vi "joe_send_message.vi"(4 "write buffer":string, 7 "source":string, 8 "write mode (set END:0)":i32(ring) items=["send EOI with last character of string", "append CR to string and send EOI with CR", "append LF to string and send EOI with LF", "append CR LF to string and send EOI with LF", "append CR to string but do not send EOI", "append LF to string but do not send EOI", "append CR LF to string but do not send EOI", "do not send EOI"], 9 "error in":errorcluster) -> (1 "byte count":i32, 5 "status":bool[](array[boolean]), 6 "error out":errorcluster)   [LabVIEW 2011]
doc: "Sends a string to a message based VXI instrument. In order to communicate with an instrument, you must first open the instrument by running the Open VXI Instrument or running the initialize VI (initialize VIs call the Open VXI Instrument in their block diagram). Use the instrument ID generated by the Open VXI Instrument to address the specific instrument, then set the write mode and enter the string to send. If a write error occurs, error code 1230 is returned. If you fail to open the instrument, error code 1232 is returned."
panel:
  in  "VISA resource name":refnum<visa-resource-name>
  in  "[empty array]":bool[](array[boolean])
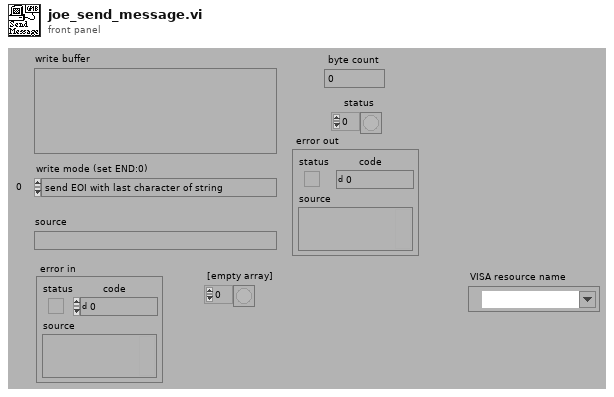
[diagram p1: front panel]
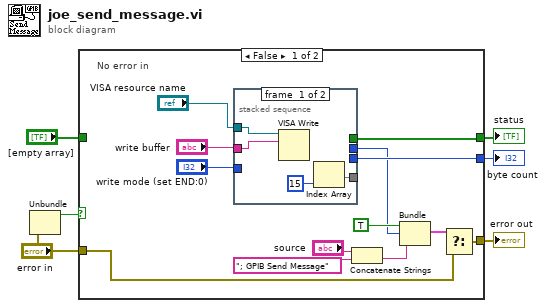
[diagram p0: block diagram]
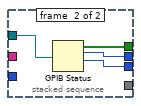
[diagram p2: hidden frame]
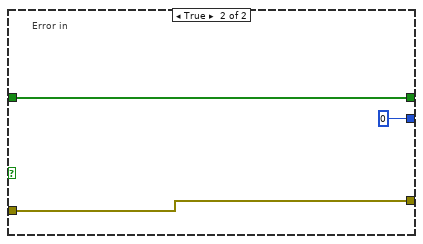
[diagram p3: hidden frame]
diagram:
  n1 = Unbundle("error in") -> ("status"=w2:bool)  [unwired: 2 out]
  n2 = case shown="False" w2 {
    tunnel: "[empty array]" -> [_ w28]
    tunnel: [w8 w28] -> w3
    tunnel: [w18 w29] -> w4
    tunnel: "error in" -> [w11 w29]
    tunnel: [w14 0] -> w6
    frame False {
      # "No error in"
      n3 = stacked-sequence {
        tunnel: [_ w26] -> w8
        tunnel: [_ w27] -> w14
        tunnel: [w22 _] -> _
        tunnel: "write mode (set END:0)" -> [_ _]
        tunnel: "write buffer" -> [w21 _]
        tunnel: [_ w25] -> w13
        tunnel: "VISA resource name" -> [w20 w24]
        frame #0 {
          n4 = VISA Write(VISA resource name=w20, write buffer=w21) -> ()  [unwired: 1 in, 3 out]
          n5 = Index Array(index=15) -> (element=w22)  [unwired: 1 in]
        }
        frame #1 {
          n6 = GPIB Status(0:w24) -> (2:w26:bool[], 3:w25:i16, 4:w27:i32)  [unwired: 1 in, 1 out]
        }
      }
      n7 = Concatenate Strings("source", "; GPIB Send Message") -> (w12:string)
      n8 = Bundle(TRUE, "GPIB error"=w13, w12) -> (w19:cluster{bool, "GPIB error":i16, string})  [unwired: 1 in]
      n9 = Select(t=w19, f=w11) -> (s? t:f=w18:errorcluster)  [unwired: 1 in]
    }
    frame True {
      # "Error in"
    }
  }
  "status" <- w3
  "error out" <- w4
  "byte count" <- w6
